vi "Read Root Model Enqueuer.vi"(11 "IViewModel In":refnum<class "IViewModel.lvclass">) -> (2 "Model Enqueuer":refnum<class "Message Enqueuer.lvclass">)   [LabVIEW 2020, in "MVA Framework.lvlib" / "IViewModel.lvlib" / "IViewModel.lvclass"]
doc: "读取根模型消息队列"
uses:
  IViewModel.lvclass
  <vilib>/ActorFramework/Message Enqueuer/Message Enqueuer.lvclass
  IViewModel.lvclass/IViewModel.ctl
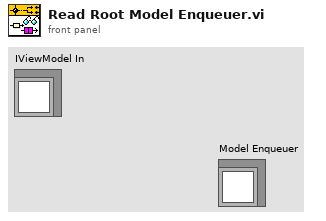
[diagram p1: front panel]
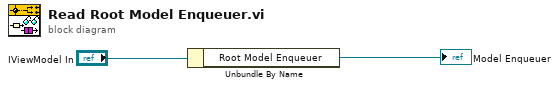
[diagram p0: block diagram]
diagram:
  n1 = Unbundle By Name("IViewModel In") -> ("Root Model Enqueuer"=→"Model Enqueuer":refnum<class "Message Enqueuer.lvclass">)
